vi "RydbergExpControl_2014.09.11_beta_2.vi"() -> ()   [LabVIEW 2013]
uses:
  AndorCamera/camera_controls.ctl
  <userlib>/atmcd32d.llb/AcquisitionMode_mode typedef.ctl
  <userlib>/atmcd32d.llb/TriggerMode_mode typedef.ctl
  6704/6704_static_voltages_control.ctl
  rydberg_state_machine_states.ctl
panel:
  out "Started in trigger snap":bool=TRUE
  out "Current Param Value":dbl
  out "Waveform Chart":dbl(graph)
  in  "Count Number?":bool
  out "Number":dbl format="%^#_6g"
  out "OD":dbl[][](graph)
  out "Atom Closeup":dbl[][](graph)
  out "Atoms - BG":dbl[][](graph)
  out "Array":dbl[](array[numeric])
  out "Background Image":dbl[][](graph)
  out "Atom Image":dbl[][](graph)
  in  "Tab Control":T1(tab)
  in  "Trigger Snap Mode":bool
  out "Camera Ready":bool
  in  "Scan Name":string
  in  "Raw_Data Folder":path
  out "Exp Running":bool
  in  "PB Instruction Time To Change":i32
  in  "Static Channel To Change":i32
  in  "Step Size":dbl min=1e-06
  in  "Final Value":dbl
  in  "Initial Value":dbl
  in  "Shutdown Experiment":bool
  in  "Start Experiment":bool
  in  "Instructions":T2(array[cluster])=[{"Instruct Data"=0, "Op Code"=0, "Flags"=[TRUE, FALSE, FALSE, FALSE, FALSE, FALSE, FALSE, FALSE, FALSE, FALSE, FALSE, FALSE, FALSE, FALSE, FALSE, FALSE, FALSE, FALSE, FALSE, FALSE, FALSE, FALSE, FALSE, FALSE], "Comments"="", "Time (s)"=0.1}, {"Instruct Data"=0, "Op Code"=0, "Flags"=[FALSE, FALSE, FALSE, FALSE, FALSE, FALSE, FALSE, FALSE, FALSE, FALSE, FALSE, FALSE, FALSE, FALSE, FALSE, FALSE, FALSE, FALSE, FALSE, FALSE, FALSE, FALSE, FALSE, FALSE], "Comments"="", "Time (s)"=0.1}, {"Instruct Data"=0, "Op Code"=0, "Flags"=[TRUE, FALSE, FALSE, FALSE, FALSE, FALSE, FALSE, FALSE, FALSE, FALSE, FALSE, FALSE, FALSE, FALSE, FALSE, FALSE, FALSE, FALSE, FALSE, FALSE, FALSE, FALSE, FALSE, FALSE], "Comments"="", "Time (s)"=0.1}, {"Instruct Data"=0, "Op Code"=6, "Flags"=[FALSE, FALSE, FALSE, FALSE, FALSE, FALSE, FALSE, FALSE, FALSE, FALSE, FALSE, FALSE, FALSE, FALSE, FALSE, FALSE, FALSE, FALSE, FALSE, FALSE, FALSE, FALSE, FALSE, FALSE], "Comments"="", "Time (s)"=0.1}] {"Time (s)" format="%.3p"; "Op Code" items=["Continue", "Stop", "Loop", "End Loop", "JSR", "RTS", "Branch", "Long Delay", "Wait"]}
  in  "What To Change":enum16{"PulseBlaster", "Static Voltage"}(ring)=enum."Static Voltage"
  out "Scan Progress":dbl(slide) caption="Slide" scale=0.0..100.0
  out "Camera Information":T3 {"VS Speed (us)" format="%.2f"}
  in  "Acquisition Parameters":T4={"Acquisition Mode"=enum."Kinetics", "Trigger Mode"=enum."External", "Frame \nTransfer"=FALSE, "Exposure Time (s)"=0.0001, "Accumulation Cycle Time (s)"=0.0, "# Accumulations"=1, "# Kinetics"=2, "Kinetic Cycle Time (s)"=0.0, "Horizontal Bin Size"=1, "Vertical Bin Size"=1} {"Vertical Bin Size" min=1; "Horizontal Bin Size" min=1; "Kinetic Cycle Time (s)" format="%.2f"; "# Kinetics" min=1; "# Accumulations" min=1; "Accumulation Cycle Time (s)" format="%.2f"; "Exposure Time (s)" format="%.2e"}
  out "Calcualted Times":T7 {"Kinetic" format="%.4f"; "Accumulate" format="%.4f"; "Exposure" format="%.4f"}
  in  "Red MOT 87 Inputs":T8={"Active Device"="6733_Red_87", "Active Channels"=[TRUE, FALSE, FALSE, FALSE, FALSE, FALSE, FALSE, FALSE], "Waveform Parameters"=[[{"Functional Form"=enum."Polynomial", "Start Voltage"=0.0, "End Voltage"=0.0, "Time"=0.0, "Degree"=1, "Sample Rate"=0.0}, {"Functional Form"=enum."Exponential", "Start Voltage"=0.0, "End Voltage"=0.0, "Time"=0.0, "Degree"=1, "Sample Rate"=0.0}, {"Functional Form"=enum."Exponential", "Start Voltage"=0.0, "End Voltage"=0.0, "Time"=0.0, "Degree"=1, "Sample Rate"=0.0}, {"Functional Form"=enum."Exponential", "Start Voltage"=0.0, "End Voltage"=0.0, "Time"=0.0, "Degree"=1, "Sample Rate"=0.0}, {"Functional Form"=enum."Exponential", "Start Voltage"=0.0, "End Voltage"=0.0, "Time"=0.0, "Degree"=1, "Sample Rate"=0.0}, {"Functional Form"=enum."Exponential", "Start Voltage"=0.0, "End Voltage"=0.0, "Time"=0.0, "Degree"=1, "Sample Rate"=0.0}], [{"Functional Form"=enum."Exponential", "Start Voltage"=0.0, "End Voltage"=0.0, "Time"=0.0, "Degree"=1, "Sample Rate"=0.0}, {"Functional Form"=enum."Exponential", "Start Voltage"=0.0, "End Voltage"=0.0, "Time"=0.0, "Degree"=1, "Sample Rate"=0.0}, {"Functional Form"=enum."Exponential", "Start Voltage"=0.0, "End Voltage"=0.0, "Time"=0.0, "Degree"=1, "Sample Rate"=0.0}, {"Functional Form"=enum."Exponential", "Start Voltage"=0.0, "End Voltage"=0.0, "Time"=0.0, "Degree"=1, "Sample Rate"=0.0}, {"Functional Form"=enum."Exponential", "Start Voltage"=0.0, "End Voltage"=0.0, "Time"=0.0, "Degree"=1, "Sample Rate"=0.0}, {"Functional Form"=enum."Exponential", "Start Voltage"=0.0, "End Voltage"=0.0, "Time"=0.0, "Degree"=1, "Sample Rate"=0.0}], [{"Functional Form"=enum."Exponential", "Start Voltage"=0.0, "End Voltage"=0.0, "Time"=0.0, "Degree"=1, "Sample Rate"=0.0}, {"Functional Form"=enum."Exponential", "Start Voltage"=0.0, "End Voltage"=0.0, "Time"=0.0, "Degree"=1, "Sample Rate"=0.0}, {"Functional Form"=enum."Exponential", "Start Voltage"=0.0, "End Voltage"=0.0, "Time"=0.0, "Degree"=1, "Sample Rate"=0.0}, {"Functional Form"=enum."Exponential", "Start Voltage"=0.0, "End Voltage"=0.0, "Time"=0.0, "Degree"=1, "Sample Rate"=0.0}, {"Functional Form"=enum."Exponential", "Start Voltage"=0.0, "End Voltage"=0.0, "Time"=0.0, "Degree"=1, "Sample Rate"=0.0}, {"Functional Form"=enum."Exponential", "Start Voltage"=0.0, "End Voltage"=0.0, "Time"=0.0, "Degree"=1, "Sample Rate"=0.0}], [{"Functional Form"=enum."Exponential", "Start Voltage"=0.0, "End Voltage"=0.0, "Time"=0.0, "Degree"=1, "Sample Rate"=0.0}, {"Functional Form"=enum."Exponential", "Start Voltage"=0.0, "End Voltage"=0.0, "Time"=0.0, "Degree"=1, "Sample Rate"=0.0}, {"Functional Form"=enum."Exponential", "Start Voltage"=0.0, "End Voltage"=0.0, "Time"=0.0, "Degree"=1, "Sample Rate"=0.0}, {"Functional Form"=enum."Exponential", "Start Voltage"=0.0, "End Voltage"=0.0, "Time"=0.0, "Degree"=1, "Sample Rate"=0.0}, {"Functional Form"=enum."Exponential", "Start Voltage"=0.0, "End Voltage"=0.0, "Time"=0.0, "Degree"=1, "Sample Rate"=0.0}, {"Functional Form"=enum."Exponential", "Start Voltage"=0.0, "End Voltage"=0.0, "Time"=0.0, "Degree"=1, "Sample Rate"=0.0}], [{"Functional Form"=enum."Exponential", "Start Voltage"=0.0, "End Voltage"=0.0, "Time"=0.0, "Degree"=1, "Sample Rate"=0.0}, {"Functional Form"=enum."Exponential", "Start Voltage"=0.0, "End Voltage"=0.0, "Time"=0.0, "Degree"=1, "Sample Rate"=0.0}, {"Functional Form"=enum."Exponential", "Start Voltage"=0.0, "End Voltage"=0.0, "Time"=0.0, "Degree"=1, "Sample Rate"=0.0}, {"Functional Form"=enum."Exponential", "Start Voltage"=0.0, "End Voltage"=0.0, "Time"=0.0, "Degree"=1, "Sample Rate"=0.0}, {"Functional Form"=enum."Exponential", "Start Voltage"=0.0, "End Voltage"=0.0, "Time"=0.0, "Degree"=1, "Sample Rate"=0.0}, {"Functional Form"=enum."Exponential", "Start Voltage"=0.0, "End Voltage"=0.0, "Time"=0.0, "Degree"=1, "Sample Rate"=0.0}], [{"Functional Form"=enum."Exponential", "Start Voltage"=0.0, "End Voltage"=0.0, "Time"=0.0, "Degree"=1, "Sample Rate"=0.0}, {"Functional Form"=enum."Exponential", "Start Voltage"=0.0, "End Voltage"=0.0, "Time"=0.0, "Degree"=1, "Sample Rate"=0.0}, {"Functional Form"=enum."Exponential", "Start Voltage"=0.0, "End Voltage"=0.0, "Time"=0.0, "Degree"=1, "Sample Rate"=0.0}, {"Functional Form"=enum."Exponential", "Start Voltage"=0.0, "End Voltage"=0.0, "Time"=0.0, "Degree"=1, "Sample Rate"=0.0}, {"Functional Form"=enum."Exponential", "Start Voltage"=0.0, "End Voltage"=0.0, "Time"=0.0, "Degree"=1, "Sample Rate"=0.0}, {"Functional Form"=enum."Exponential", "Start Voltage"=0.0, "End Voltage"=0.0, "Time"=0.0, "Degree"=1, "Sample Rate"=0.0}], [{"Functional Form"=enum."Exponential", "Start Voltage"=0.0, "End Voltage"=0.0, "Time"=0.0, "Degree"=1, "Sample Rate"=0.0}, {"Functional Form"=enum."Exponential", "Start Voltage"=0.0, "End Voltage"=0.0, "Time"=0.0, "Degree"=1, "Sample Rate"=0.0}, {"Functional Form"=enum."Exponential", "Start Voltage"=0.0, "End Voltage"=0.0, "Time"=0.0, "Degree"=1, "Sample Rate"=0.0}, {"Functional Form"=enum."Exponential", "Start Voltage"=0.0, "End Voltage"=0.0, "Time"=0.0, "Degree"=1, "Sample Rate"=0.0}, {"Functional Form"=enum."Exponential", "Start Voltage"=0.0, "End Voltage"=0.0, "Time"=0.0, "Degree"=1, "Sample Rate"=0.0}, {"Functional Form"=enum."Exponential", "Start Voltage"=0.0, "End Voltage"=0.0, "Time"=0.0, "Degree"=1, "Sample Rate"=0.0}], [{"Functional Form"=enum."Exponential", "Start Voltage"=0.0, "End Voltage"=0.0, "Time"=0.0, "Degree"=1, "Sample Rate"=0.0}, {"Functional Form"=enum."Exponential", "Start Voltage"=0.0, "End Voltage"=0.0, "Time"=0.0, "Degree"=1, "Sample Rate"=0.0}, {"Functional Form"=enum."Exponential", "Start Voltage"=0.0, "End Voltage"=0.0, "Time"=0.0, "Degree"=1, "Sample Rate"=0.0}, {"Functional Form"=enum."Exponential", "Start Voltage"=0.0, "End Voltage"=0.0, "Time"=0.0, "Degree"=1, "Sample Rate"=0.0}, {"Functional Form"=enum."Exponential", "Start Voltage"=0.0, "End Voltage"=0.0, "Time"=0.0, "Degree"=1, "Sample Rate"=0.0}, {"Functional Form"=enum."Exponential", "Start Voltage"=0.0, "End Voltage"=0.0, "Time"=0.0, "Degree"=1, "Sample Rate"=1.0}]], "Active Phases"=[TRUE, FALSE, FALSE, FALSE, FALSE, FALSE], "Phase Times"=[0.001], "Trigger Channel"="/6733_Red_87/PFI0"} {"Phase Times" format="%.0p"; "Waveform Parameters"."Degree" min=1}
  in  "6704 Static Voltage Settings":T9={"Device Name"="6704_Static", "Voltages"=[5.0, 0.0, 0.0, 0.0, 0.0, 0.0, 0.0, 0.0, 0.0, 0.0, 0.0, 0.0, 0.0, 0.0, 0.0, 0.0]}
  out "Andor Initialization Error Codes":T10
  out "Acq. Error Codes":T11
  out "Tree":string(tree)
  # "(1) 461 MOT beams"
  # "(2) Imaging AOM 1"
  # "(3) Imaging AOM 2"
  # "(4) Camera"
  # "(5) Zeeman shutter"
  # "(6) Repumper shutter"
  # "(7) 461 MOT coils"
  # "(8) 689 MOT coils"
  # "(9) 87 Sr Red MOT Trig"
  # "(10) ??? Shutter"
  # "(11) Red AOM"
  # "(12) Sat Abs Current Switch"
  # "(13) Zeeman MOSFET"
  # "1"
  # "2"
  # "3"
  # "4"
  # "5"
  # "6"
  # "7"
  # "8"
  # "9"
  # "10"
  # "11"
  # "12"
  # "13"
  # "14"
  # "15"
  # "16"
  # "17"
  # "18"
  # "19"
  # "20"
  # "21"
  # "22"
  # "23"
  # "24"
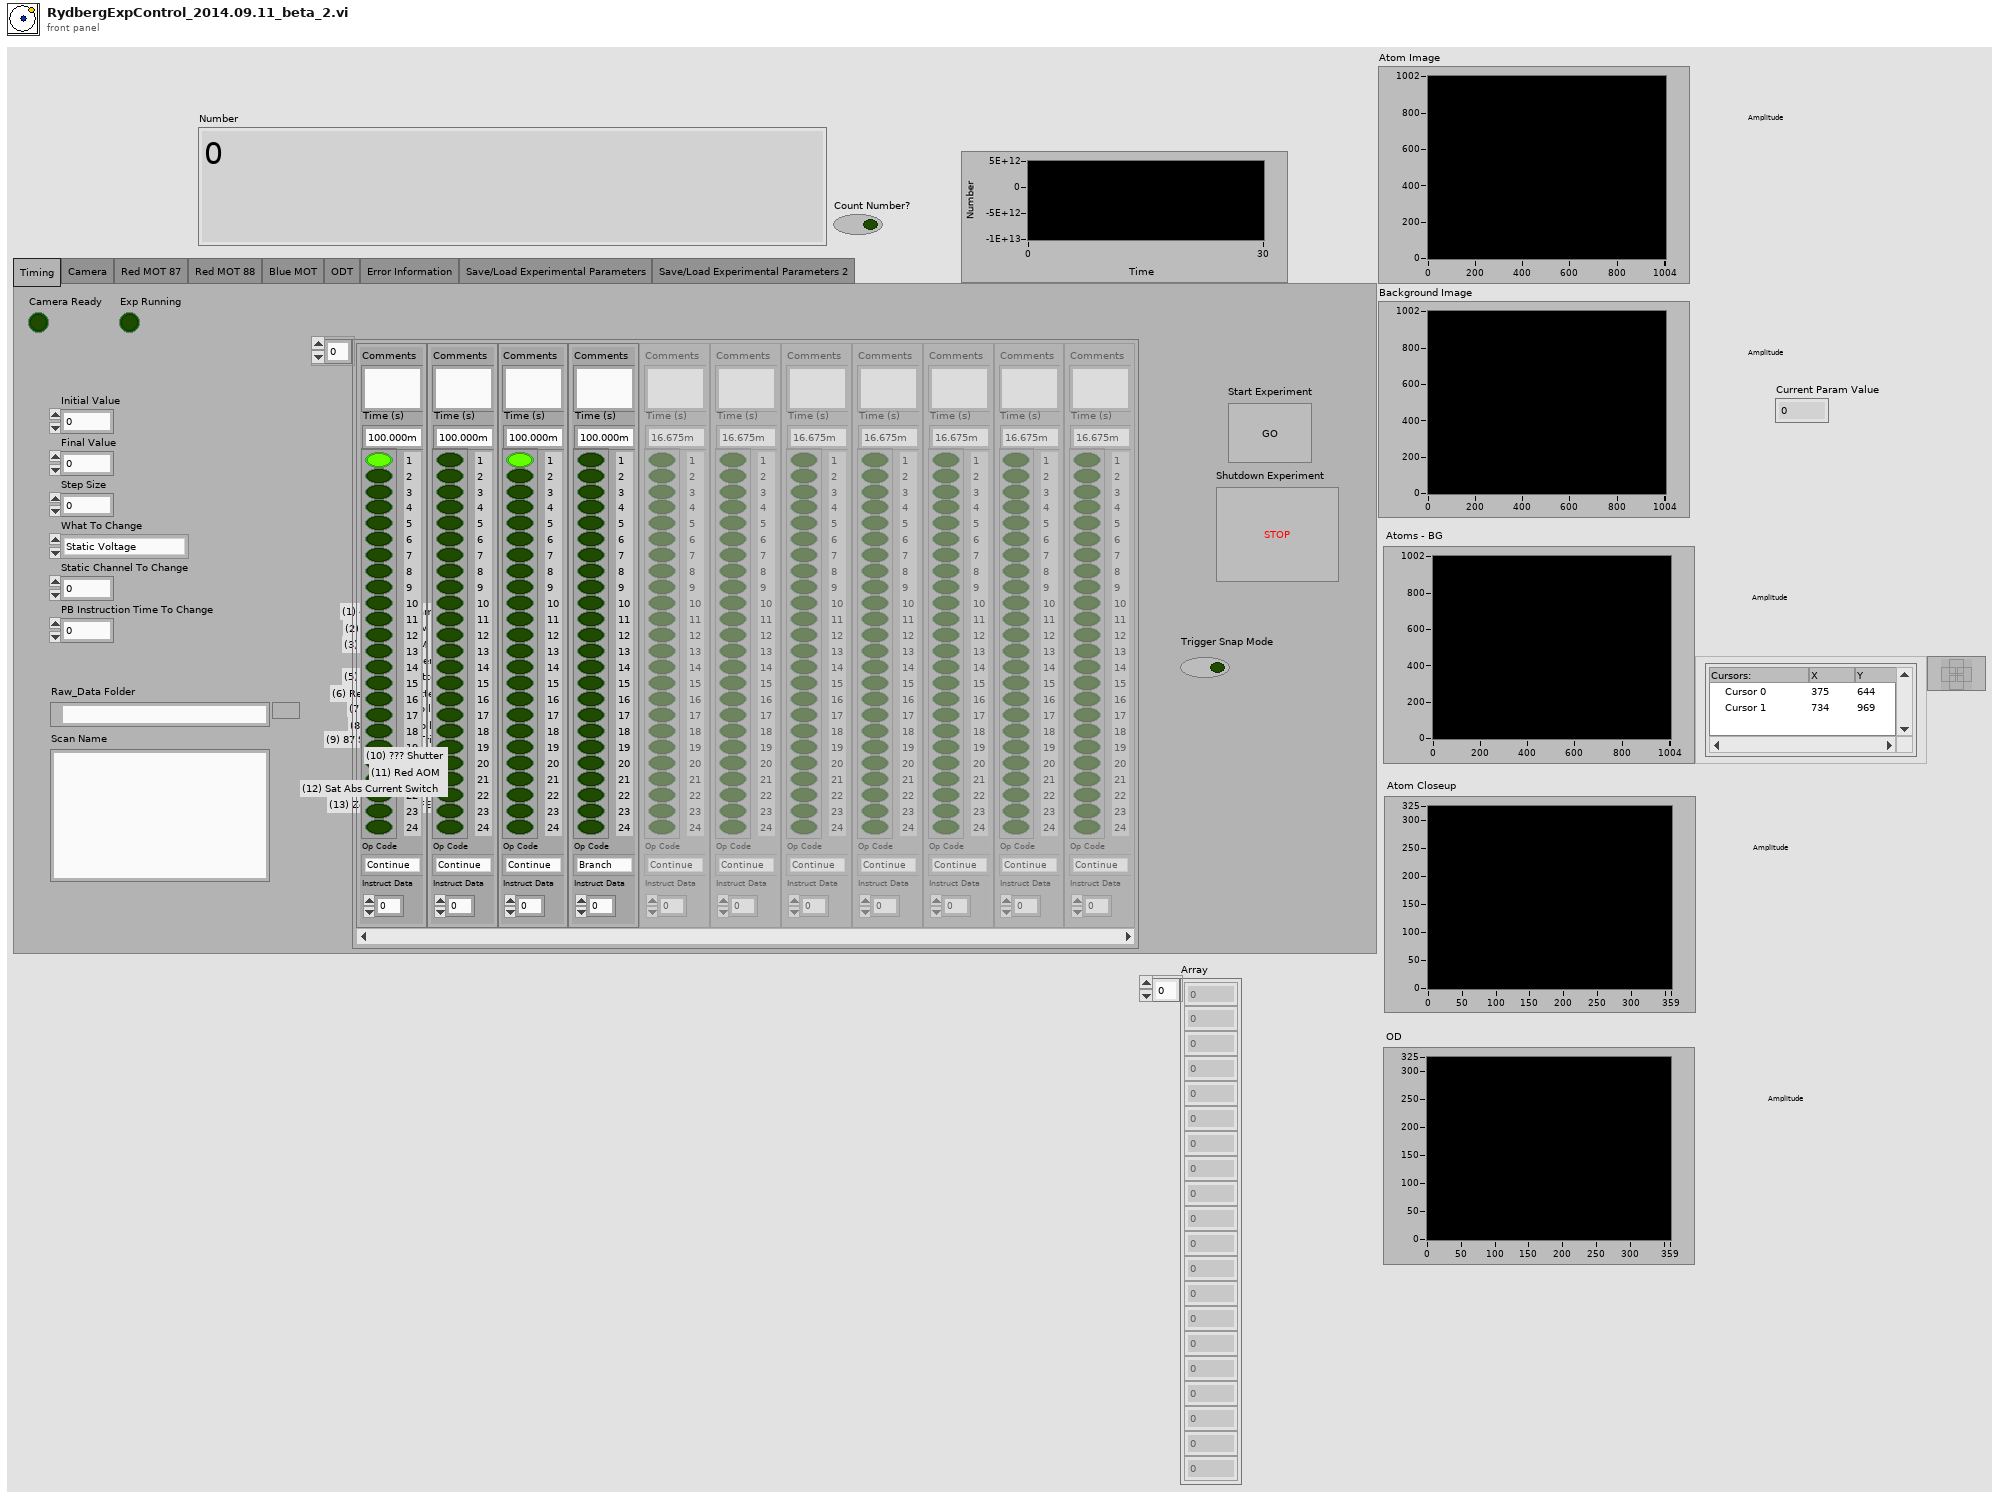
[diagram p1: front panel]
types:
  T1 = enum32{"Timing", "Camera", "Red MOT 87", "Red MOT 88", "Blue MOT", "ODT", "Error Information", "Save/Load Experimental Parameters", "Save/Load Experimental Parameters 2"}
  T2 = cluster{"Instruct Data":i32, "Op Code":i32, "Flags":bool[], "Comments":string, "Time (s)":dbl}[]
  T3 = cluster{"xpixels":i32, "ypixels":i32, "# VS Speeds":i32, "VS Speed (us)":sgl, "Temperature Stable":bool, "Temperature (C)":i32}
  T4 = typedef "camera_controls.ctl" = cluster{"Acquisition Mode":T5, "Trigger Mode":T6, "Frame \nTransfer":bool, "Exposure Time (s)":sgl, "Accumulation Cycle Time (s)":sgl, "# Accumulations":i32, "# Kinetics":i32, "Kinetic Cycle Time (s)":sgl, "Horizontal Bin Size":i32, "Vertical Bin Size":i32}
  T5 = typedef "AcquisitionMode_mode typedef.ctl" = enum16{"Reserved (0)", "Single Scan", "Accumulate", "Kinetics", "Fast Kinetics", "Run Till Abort", "Reserved (6)", "Reserved (7)", "Reserved (8)", "Time Delayed Integration"}
  T6 = typedef "TriggerMode_mode typedef.ctl" = enum16{"Internal", "External", "N/A (2)", "N/A (3)", "N/A (4)", "N/A (5)", "External Start", "External Exposure (Bulb)", "N/A (8)", "External FVB EM", "Software", "N/A (11)", "External Charge Shifting"}
  T7 = cluster{"Exposure":sgl, "Accumulate":sgl, "Kinetic":sgl}
  T8 = cluster{"Active Device":string, "Active Channels":bool[], "Waveform Parameters":cluster{"Functional Form":enum16{"Polynomial", "Exponential"}, "Start Voltage":dbl, "End Voltage":dbl, "Time":dbl, "Degree":i8, "Sample Rate":dbl}[][], "Active Phases":bool[], "Phase Times":dbl[], "Trigger Channel":tag}
  T9 = typedef "6704_static_voltages_control.ctl" = cluster{"Device Name":string, "Voltages":dbl[]}
  T10 = cluster{"Initalize Error Code":u32, "GetDetector Error Code":u32, "Get#VSSpeeds Error Code":u32, "Set VS Speed Error":u32, "CoolerOn Error Code":u32, "GetTemperature Error Code":u32, "Shutdown Error Code":u32}
  T11 = cluster{"Set Acq. Mode Error":u32, "Set Trigger Mode Error":u32, "Set FT Error Code":u32, "Set Exposure Time Error Code":u32, "Set Accum Time Error":u32, "Set # Accum Error":u32, "Set # Kinetics Error":u32, "SetKinCycleTime Error":u32}
  T12 = typedef "rydberg_state_machine_states.ctl" = enum16{"Initialize", "Idle", "Experiment Running", "Trigger Snap Mode", "Scan Mode", "Load Experiment", "Shutdown"}
  T13 = cluster{"6704 Static Voltage Settings":T9, "Instructions":cluster{"Instruct Data":i32, "Op Code":i32, "Flags":bool[], "Comments":string, "Time (s)":dbl}[], "Red MOT 87 Inputs":cluster{"Active Device":string, "Active Channels":bool[], "Waveform Parameters":cluster{"Functional Form":enum16{"Polynomial", "Exponential"}, "Start Voltage":dbl, "End Voltage":dbl, "Time":dbl, "Degree":i8, "Sample Rate":dbl}[][], "Active Phases":bool[], "Phase Times":dbl[], "Trigger Channel":tag}}
  T14 = typedef "LVCursorListTypeDef.ctl" = cluster{"Name":string, "Color":u32, "Style":u8, "Point Style":u8, "Name Visible":bool, "Allow Drag":bool, "Cursor Mode":u32, "Plot":i32, "Index":i32, "Position":cluster{"X":dbl, "Y":dbl}, "X Scale":u32, "Y Scale":u32, "Watch Plots":i32[], "Watch All Plots":bool, "Plot Area":i32, "Label Offset":cluster{"X":dbl, "Y":dbl}}[]
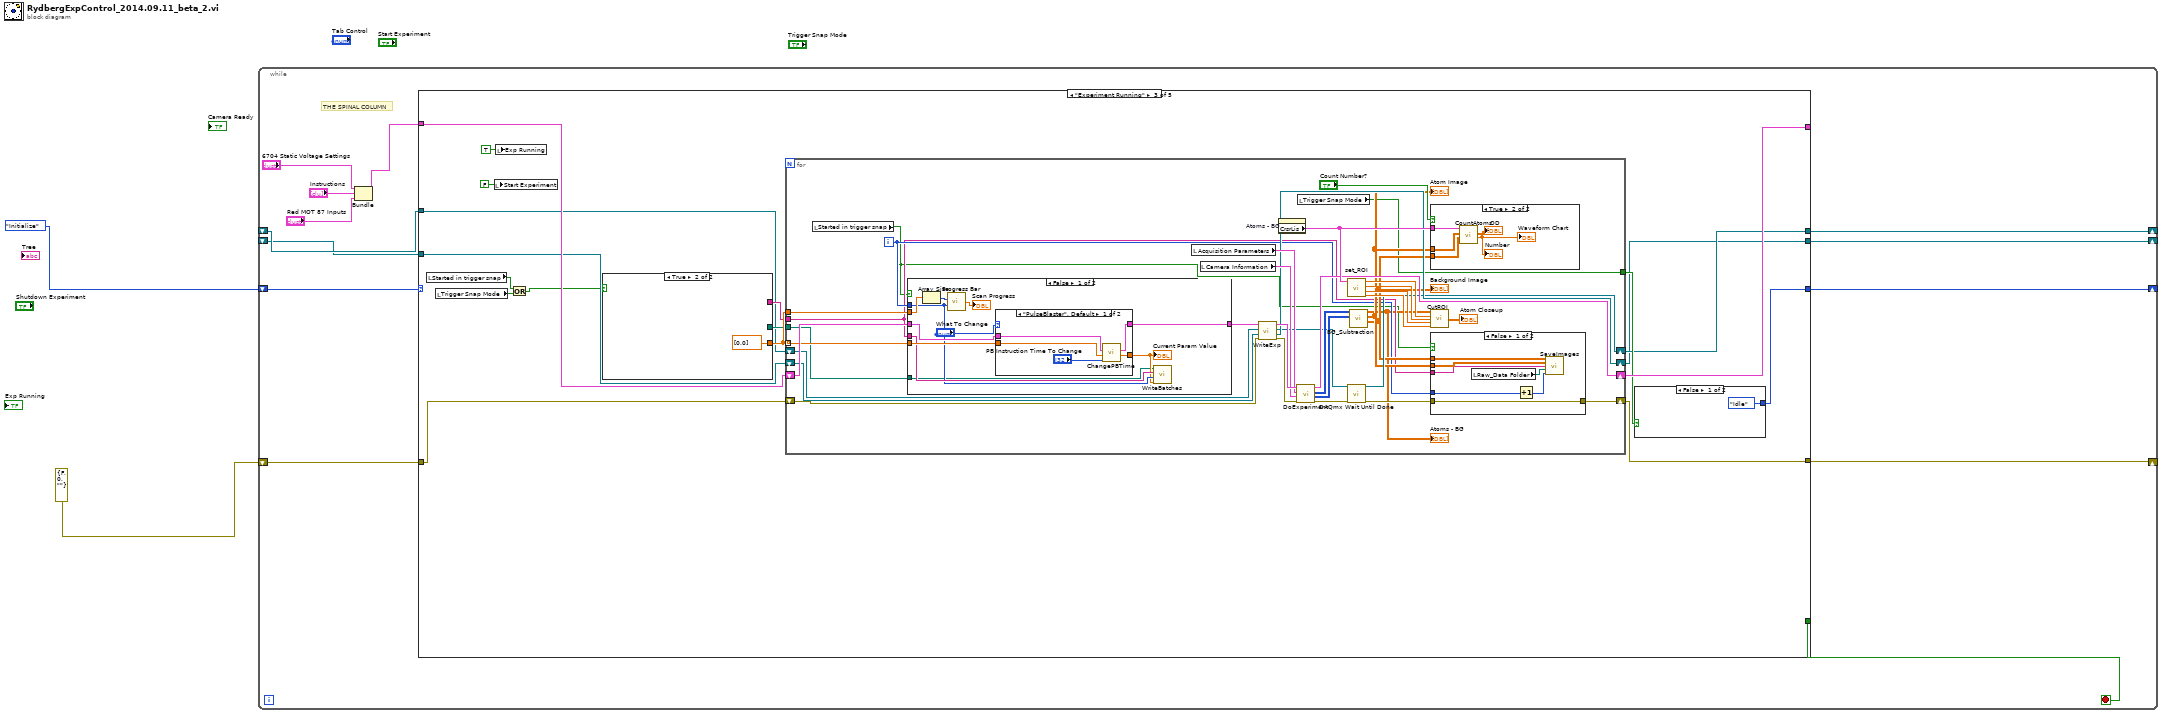
[diagram p0: block diagram]
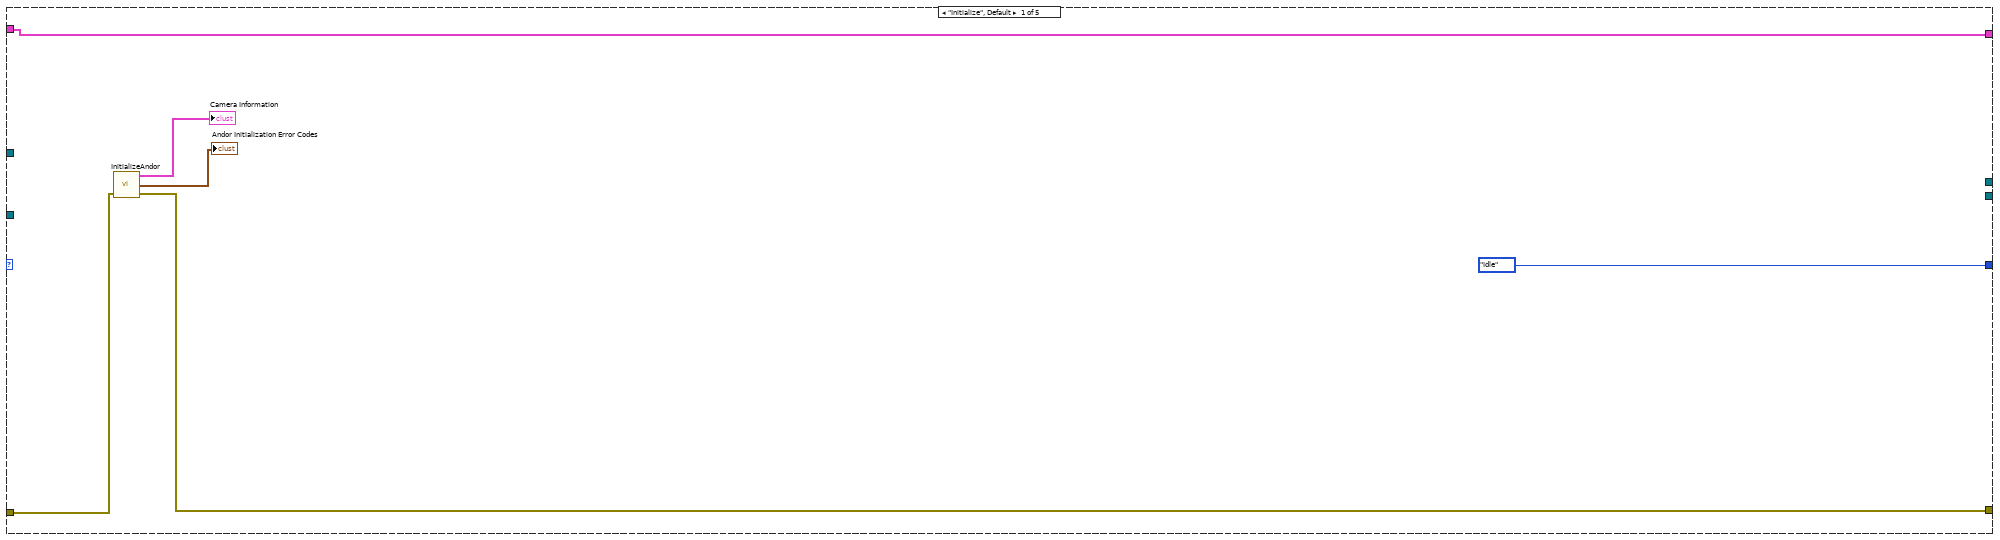
[diagram p2: hidden frame]
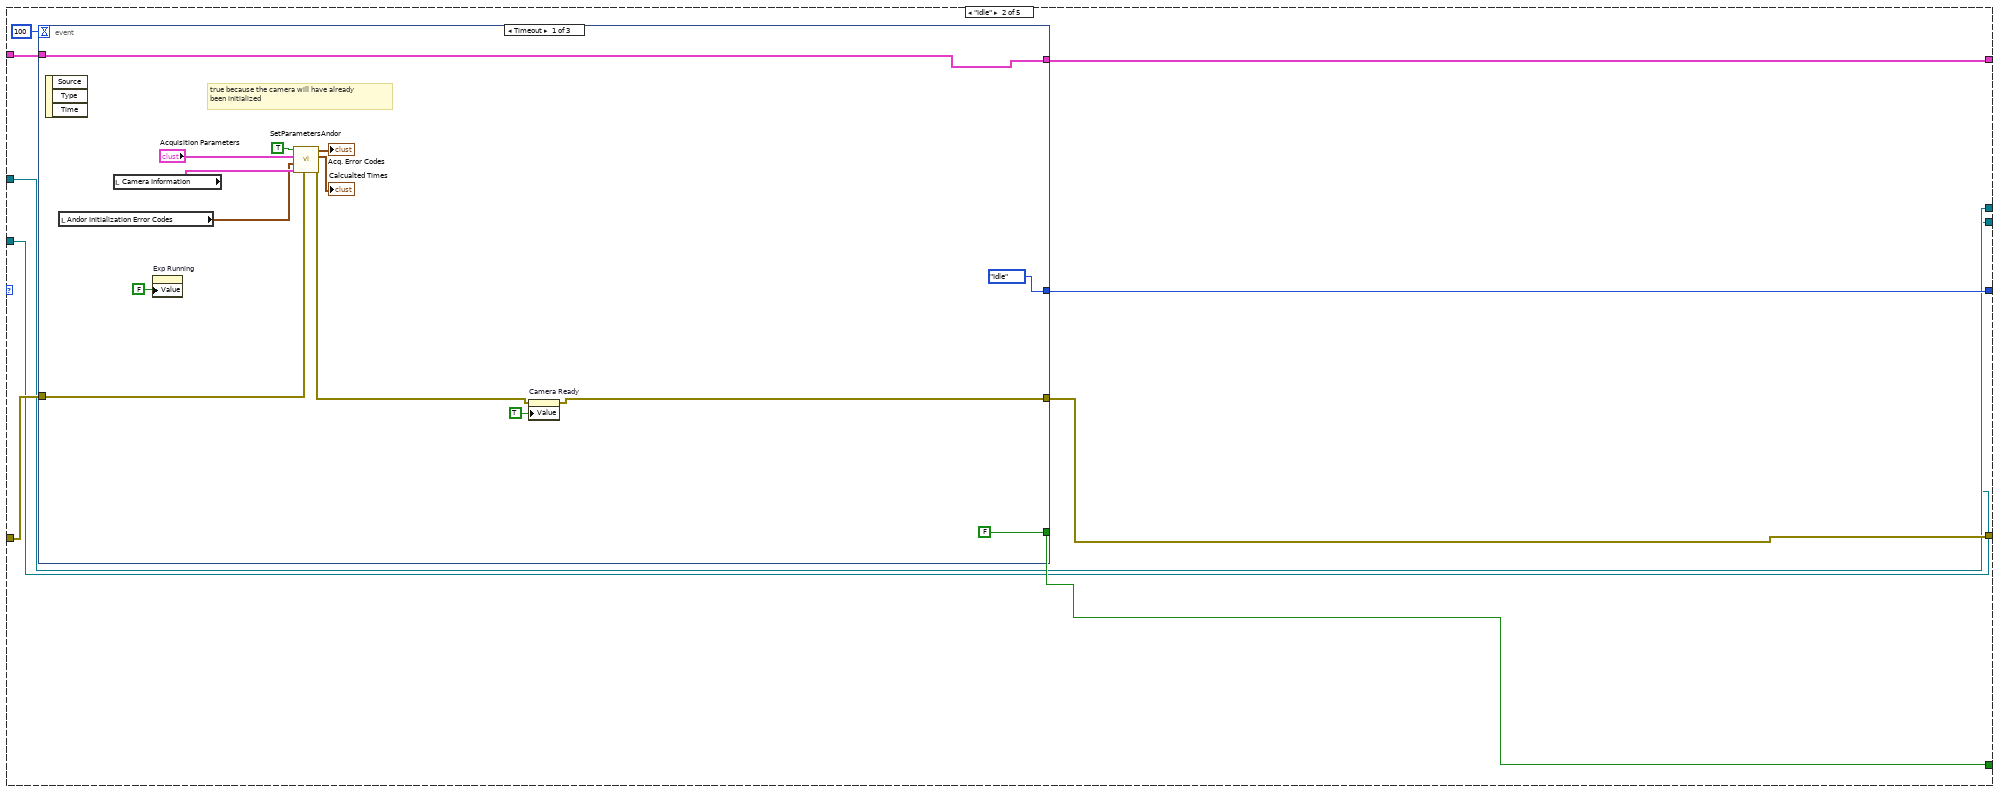
[diagram p3: hidden frame]
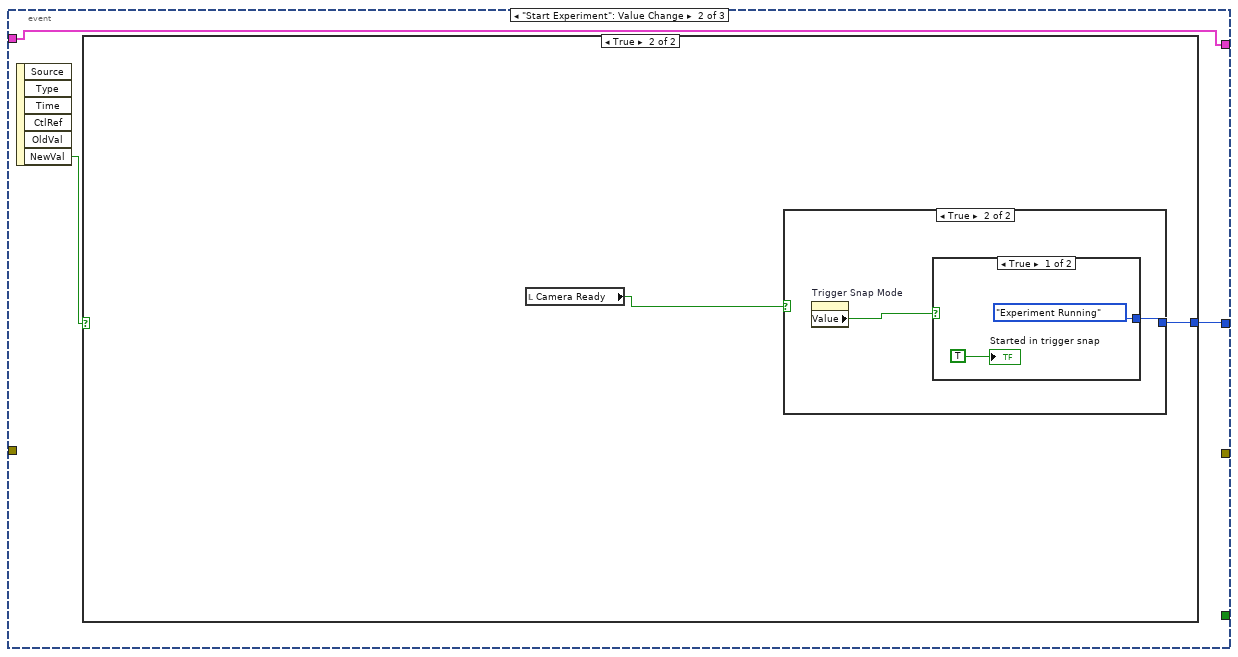
[diagram p4: hidden frame]
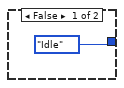
[diagram p5: hidden frame]
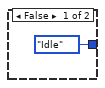
[diagram p6: hidden frame]
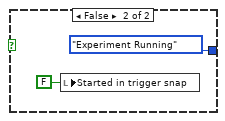
[diagram p7: hidden frame]
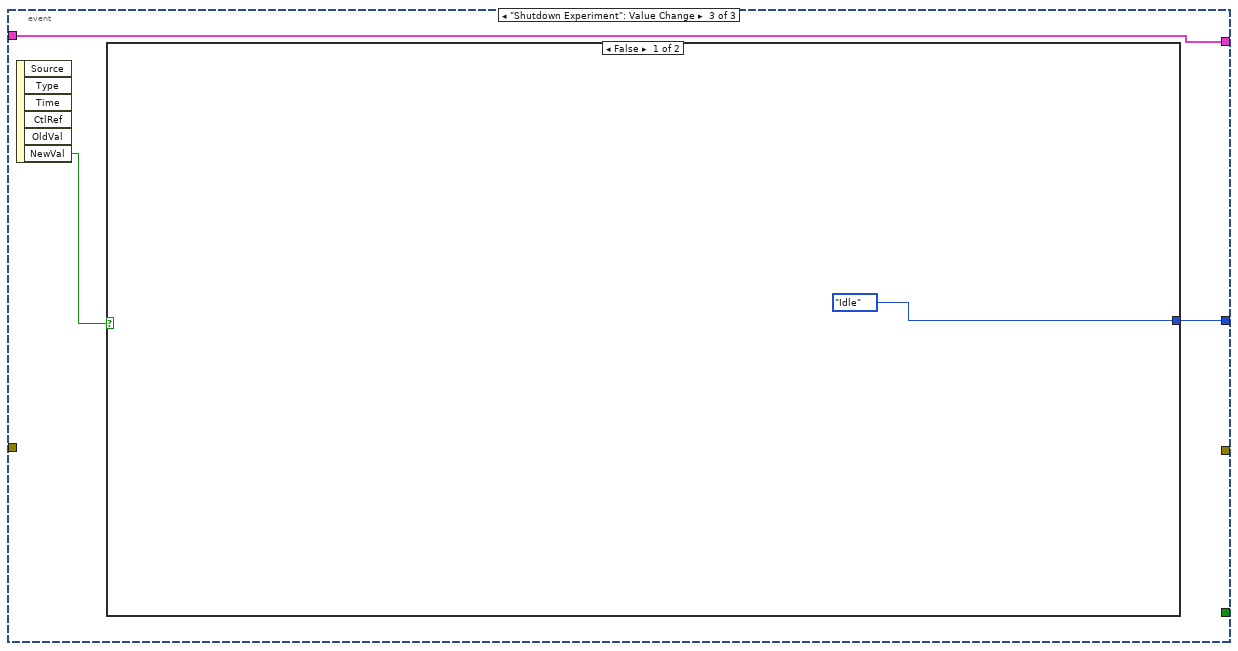
[diagram p8: hidden frame]
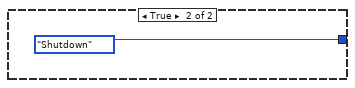
[diagram p9: hidden frame]
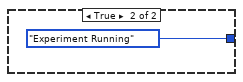
[diagram p10: hidden frame]
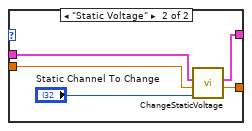
[diagram p13: hidden frame]
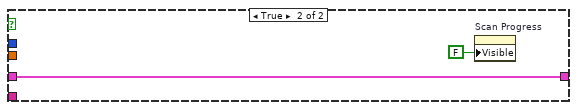
[diagram p14: hidden frame]
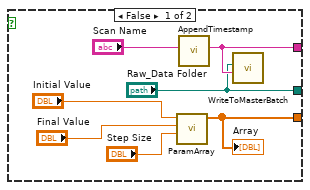
[diagram p15: hidden frame]
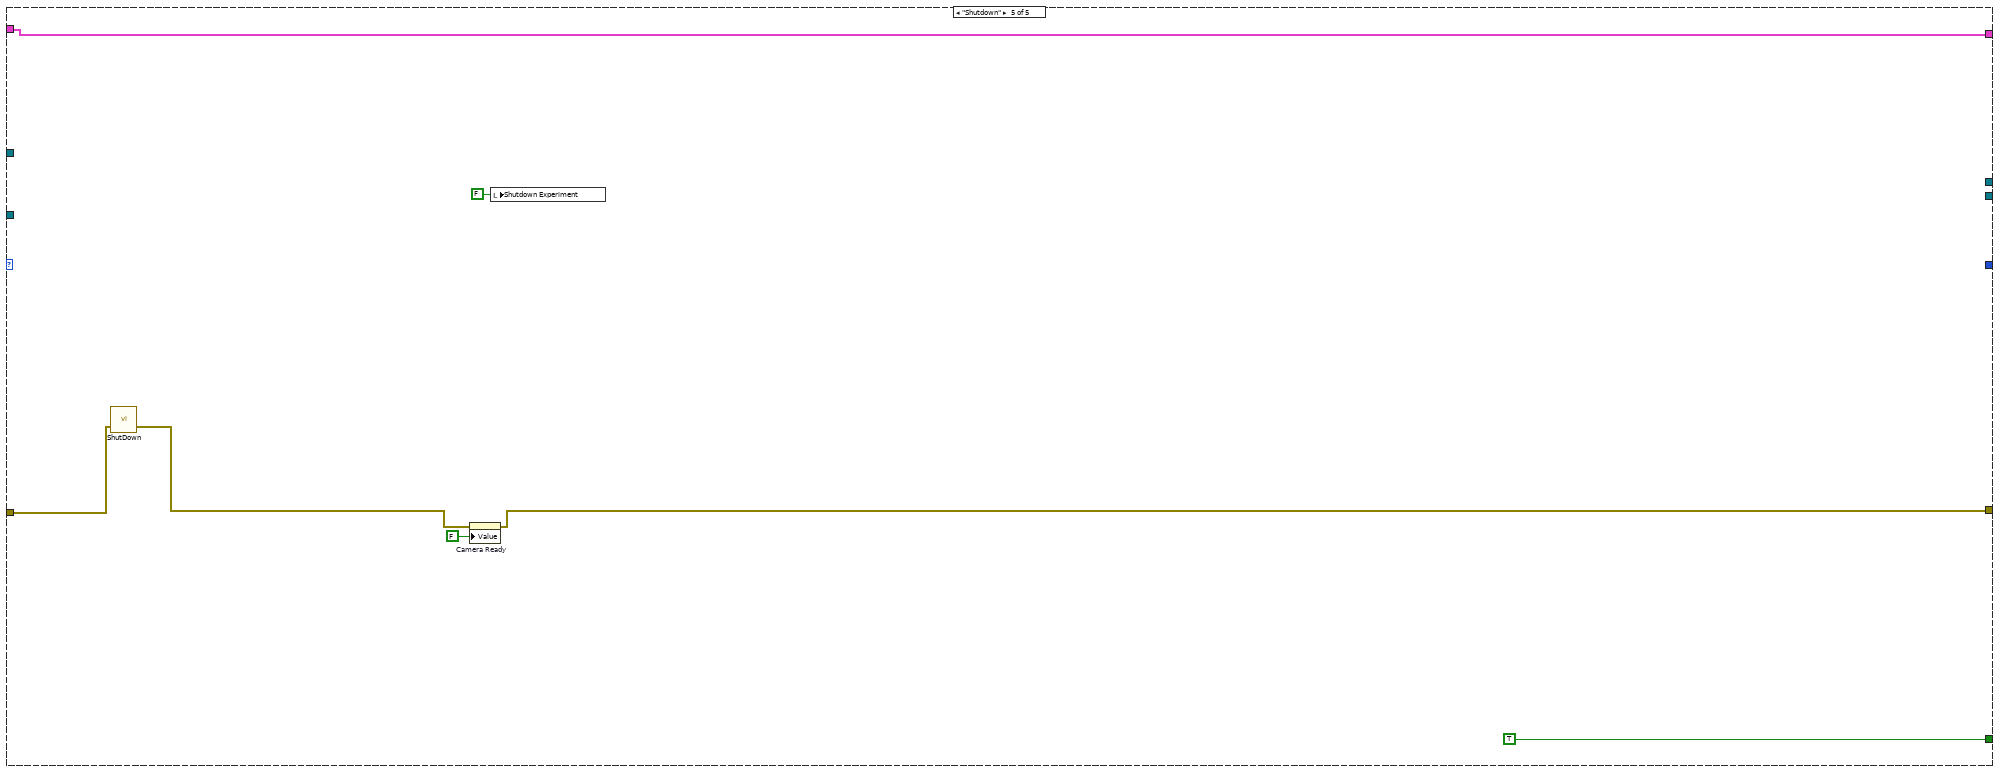
[diagram p17: hidden frame]
diagram:
  n1 = while {
    shift-right: [w12] -> _
    shift-left: rydberg_state_machine_states."Initialize" -> [w15]
    shift-right: [w13] -> _
    shift-left: errorcluster {"status"=FALSE, "code"=0, "source"=""} ("error constant") -> [w14]
    shift-right: [w6] -> _
    shift-left: _ -> [w5]
    shift-right: [w4] -> _
    shift-left: _ -> [w3]
    stop <- w11 stop-if-true
    # "THE SPINAL COLUMN"
    n2 = Bundle("6704 Static Voltage Settings"="6704 Static Voltage Settings", "Instructions"="Instructions", "Red MOT 87 Inputs"="Red MOT 87 Inputs") -> (w7:T13)  [unwired: 1 in]
    n3 = case shown="\"Experiment Running\"" w15 {
      tunnel: w14 -> [w21 w30 w78 _ w169]
      tunnel: [w18 w26 w76 _ w164] -> w13
      tunnel: [rydberg_state_machine_states."Idle" w28 w71 _ _] -> w12
      tunnel: [_ w27 _ _ TRUE] -> w11
      tunnel: [w16 w25 w73 w162 w166] -> _
      tunnel: w7 -> [w16 w24 w79 w162 w166]
      tunnel: [_ w23 w70 _ _] -> w6
      tunnel: w5 -> [_ w23 w67 _ _]
      tunnel: [_ w22 w69 _ _] -> w4
      tunnel: w3 -> [_ w22 w68 _ _]
      frame "Initialize", Default {
        n4 = call "InitializeAndor.vi"("Error In"=w21) -> ("error out"=w18:errorcluster, "Andor Initialization Error Codes"=→"Andor Initialization Error Codes":T10, "Camera Information"=→"Camera Information":T3)  [unwired: 2 in]
      }
      frame "Idle" {
        n5 = event shown="[0] Timeout" {
          selector: _ -> [_ _ _]
          dyn-events: _ -> [_ _ _]
          timeout: 100 -> [_ _ _]
          tunnel: w30 -> [w38 _ _]
          tunnel: [rydberg_state_machine_states."Idle" w46 w59] -> w28
          tunnel: [FALSE _ _] -> w27
          tunnel: [w32 _ _] -> w26
          tunnel: [w35 w45 w58] -> w25
          tunnel: w24 -> [w35 w45 w58]
          event Timeout {
            # "true because the camera will have already\nbeen initialized"
            n6 = event-data() -> ()  [unwired: 1 in, 3 out]
            n7 = local read "Andor Initialization Error Codes"() -> (w37:T10)
            n8 = local read "Camera Information"() -> (w40:T3)
            n9 = property on="Exp Running" class="Bool (strict)"("Value"=FALSE ("Exp Running")) -> ()  [unwired: 2 in, 2 out]
            n10 = call "SetParametersAndor.vi"("Error In"=w38, "Camera Information"=w40, "Andor Initialization Error Codes"=w37, "Acquisition Parameters"="Acquisition Parameters", "Pre Initialized?"=TRUE) -> ("error out"=w33:errorcluster, "Calcualted Times"=→"Calcualted Times":T7, "Acq. Error Codes"=→"Acq. Error Codes":T11)  [unwired: 4 in]
            n11 = property on="Camera Ready" class="Bool (strict)"(error in=w33, "Value"=TRUE ("Camera Ready")) -> (error out=w32:errorcluster)  [unwired: 1 in, 1 out]
          }
          event "Start Experiment": Value Change {
            n12 = event-data() -> ("NewVal"=w47:bool)  [unwired: 1 in, 5 out]
            n13 = case shown="True" w47 {
              tunnel: [rydberg_state_machine_states."Idle" w50] -> w46
              frame False {
              }
              frame True {
                n14 = local read "Camera Ready"() -> (w49:bool)
                n15 = case shown="True" w49 {
                  tunnel: [rydberg_state_machine_states."Idle" w53] -> w50
                  frame False {
                  }
                  frame True {
                    n16 = property on="Trigger Snap Mode" class="Bool (strict)"() -> ("Value"=w52:bool)  [unwired: 2 in, 2 out]
                    n17 = case shown="True" w52 {
                      tunnel: [rydberg_state_machine_states."Experiment Running" rydberg_state_machine_states."Experiment Running"] -> w53
                      frame True {
                        "Started in trigger snap" <- TRUE
                      }
                      frame False {
                        n18 = local write "Started in trigger snap"(FALSE ("Started in trigger snap")) -> ()
                      }
                    }
                  }
                }
              }
            }
          }
          event "Shutdown Experiment": Value Change {
            n19 = event-data() -> ("NewVal"=w60:bool)  [unwired: 1 in, 5 out]
            n20 = case shown="False" w60 {
              tunnel: [rydberg_state_machine_states."Idle" rydberg_state_machine_states."Shutdown"] -> w59
              frame False {
              }
              frame True {
              }
            }
          }
        }
      }
      frame "Experiment Running" {
        n21 = local read "Started in trigger snap"() -> (w64:bool)
        n22 = local read "Trigger Snap Mode"() -> (w65:bool)
        n23 = local write "Start Experiment"(FALSE ("Start Experiment")) -> ()
        n24 = local write "Exp Running"(TRUE ("Exp Running")) -> ()
        n25 = Or(x=w64, y=w65) -> (x .or. y?=w63:bool)
        n26 = case shown="True" w63 {
          tunnel: [w156 dbl[] [0.0]] -> w77
          tunnel: [w155 _] -> w75
          tunnel: ["Raw_Data Folder" _] -> w74
          frame False {
            n27 = call "ParamArray.vi"("Step Size"="Step Size", "Final Value"="Final Value", "Initial Value"="Initial Value") -> ("Array"=w156:dbl[])  [unwired: 8 in]
            "Array" <- w156
            n28 = call "AppendTimestamp.vi"("String"="Scan Name") -> ("String 2"=w155:string)  [unwired: 10 in]
            n29 = call "WriteToMasterBatch.vi"("Scan name"=w155, "Raw_Data Folder"="Raw_Data Folder") -> ()  [unwired: 10 in]
          }
          frame True {
          }
        }
        n30 = for {
          shift-right: [w100] -> w73
          shift-left: w79 -> [w117]
          tunnel: w77 -> [w116] mode=indexing
          shift-right: [w93] -> w70
          shift-left: w67 -> [w99]
          shift-right: [w97] -> w69
          shift-left: w68 -> [w98]
          tunnel: w77 -> [w96]
          shift-right: [w90] -> w76
          shift-left: w78 -> [w114]
          tunnel: w75 -> [w86]
          tunnel: w74 -> [w92]
          tunnel: [w84] -> w72
          i -> [w87]
          n31 = local read "Started in trigger snap"() -> (w83:bool)
          n32 = case shown="False" w83 {
            tunnel: w117 -> [w140 w153]
            tunnel: w116 -> [w139 _]
            tunnel: [w138 w153] -> w115
            tunnel: w87 -> [w133 _]
            tunnel: w96 -> [w137 _]
            tunnel: w86 -> [w134 _]
            tunnel: w92 -> [w131 _]
            frame False {
              n33 = Array Size(array=w137) -> (size(s)=w136:i32)
              n34 = call "Progress Bar.vi"("Total Number"=w136, "Current Number"=w133) -> ("Scan Progress"=→"Scan Progress":dbl)  [unwired: 13 in]
              n35 = case shown="\"PulseBlaster\", Default" "What To Change" {
                tunnel: w140 -> [w146 w151]
                tunnel: w139 -> [w143 w149]
                tunnel: [w145 w148] -> w138
                tunnel: [w142 w147] -> w132
                frame "PulseBlaster", Default {
                  n36 = call "ChangePBTime.vi"("Instruction to change"="PB Instruction Time To Change", "Time"=w143, "Input parameters"=w146) -> ("Time out"=w142:dbl, "output parameters"=w145:T13)  [unwired: 7 in]
                }
                frame "Static Voltage" {
                  n37 = call "ChangeStaticVoltage.vi"("Channel to change"="Static Channel To Change", "Voltage"=w149, "Parameters input"=w151) -> ("Voltage out"=w147:dbl, "Parameters Output"=w148:T13)  [unwired: 7 in]
                }
              }
              "Current Param Value" <- w132
              n38 = call "WriteBatches.vi"("Variable Parameter Value"=w132, "Image Number"=w133, "String"=w134, "Raw Data Folder"=w131) -> ()  [unwired: 8 in]
            }
            frame True {
              n39 = property on="Scan Progress" class="Slide (strict)"("Visible"=FALSE) -> ()  [unwired: 2 in, 2 out]
            }
          }
          n40 = local read "Acquisition Parameters"() -> (w111:T4)
          n41 = local read "Camera Information"() -> (w112:T3)
          n42 = call "WriteExp.vi"("error in (no error)"=w114, "Control Task In"=w98, "Waveform Task In"=w99, "Experimental Control Cluster In"=w115) -> ("error out"=w110:errorcluster, "waveform task out"=w97:refnum<k21>, "counter task out"=w95:refnum<k21>, "Experimental Control Cluster Out"=w113:T13)  [unwired: 4 in]
          n43 = property on="Atoms - BG" class="IntGraph (strict)"() -> ("CrsrLis"=w101:T14)  [unwired: 2 in, 2 out]
          n44 = call "DoExperiment.vi"("Error In"=w110, "Camera Information 2"=w112, "Acquisition Parameters"=w111, "output cluster"=w113) -> ("error out"=w94:errorcluster, "Background Image"=w109:i32[][], "Atom Image"=w108:i32[][], "output cluster 2"=w100:T13)  [unwired: 4 in]
          n45 = local read "Trigger Snap Mode"() -> (w84:bool)
          n46 = call "set_ROI.vi"("Cursor List"=w101) -> ("Row End"=w104:dbl, "RowStart"=w105:dbl, "ColEnd"=w106:dbl, "ColStart"=w107:dbl)  [unwired: 7 in]
          n47 = call <vilib>:"DAQmx Wait Until Done.vi"("task/channels in"=w95, "error in"=w94) -> ("task out"=w93:refnum<k21>, "error out"=w91:errorcluster)  [unwired: 12 in]
          n48 = call "BG_Subtraction.vi"("Background Image"=w109, "Atom Image"=w108) -> ("Background Image Out"=w88:dbl[][], "Atom Image Out"=w89:dbl[][], "Atoms - BG"=w85:dbl[][])  [unwired: 7 in]
          "Background Image" <- w88
          "Atom Image" <- w89
          "Atoms - BG" <- w85
          n49 = case shown="True" "Count Number?" {
            tunnel: w101 -> [_ w130]
            tunnel: w89 -> [_ w129]
            tunnel: w88 -> [_ w128]
            frame False {
            }
            frame True {
              n50 = call "CountAtoms.vi"("Background Image"=w128, "Atom Image"=w129, "Cursor List"=w130) -> ("Number"=→"Waveform Chart" →"Number":dbl, "OD"=→"OD":dbl[][])  [unwired: 7 in]
            }
          }
          n51 = call "CutROI.vi"("Full Image In"=w85, "Col Start"=w107, "Col End"=w106, "Row Start"=w105, "Row End"=w104) -> ("Cut Image Out"=→"Atom Closeup":dbl[][])  [unwired: 10 in]
          n52 = case shown="False" w83 {
            tunnel: [w124 w125] -> w90
            tunnel: w91 -> [w124 w125]
            tunnel: w89 -> [w122 _]
            tunnel: w88 -> [w121 _]
            tunnel: w87 -> [w119 _]
            tunnel: w86 -> [w120 _]
            frame False {
              n53 = local read "Raw_Data Folder"() -> (w123:path)
              n54 = Increment(x=w119) -> (x+1=w118:i32)
              n55 = call "SaveImages.vi"("Background Image"=w121, "Atoms Image"=w122, "Base Filename"=w120, "Raw Data Path"=w123, "ImageNumber"=w118) -> ()  [unwired: 9 in, 2 out]
            }
            frame True {
            }
          }
        }
        n56 = case shown="False" w72 {
          tunnel: [rydberg_state_machine_states."Idle" rydberg_state_machine_states."Experiment Running"] -> w71
          frame False {
          }
          frame True {
          }
        }
      }
      frame "Load Experiment" {
      }
      frame "Shutdown" {
        n57 = call <userlib>:"ShutDown.vi"("error in (no error)"=w169) -> ("error out"=w165:errorcluster)  [unwired: 1 in, 1 out]
        n58 = property on="Camera Ready" class="Bool (strict)"(error in=w165, "Value"=FALSE ("Camera Ready")) -> (error out=w164:errorcluster)  [unwired: 1 in, 1 out]
        n59 = local write "Shutdown Experiment"(FALSE ("Shutdown Experiment")) -> ()
      }
    }
  }
